vi "電池正負極設定.vi"() -> (3 "File Path":path=path "D:/battery/positive.txt")   [LabVIEW 2015]
uses:
  <vilib>/Utility/miscctls.llb/LVPointTypeDef.ctl
panel:
  in  "電池正負極陣列(輸入)":bool[](array[boolean])
  out "Enum":enum16{"一、讀取影像", "二、讀取設定檔", "三、寫入設定檔", "四、離開"}(ring)
  in  "離開":bool
  in  "寫入設定檔":bool
  in  "讀取設定檔":bool
  out "電池正負極陣列(輸出)":bool[](array[boolean])
  in  "電池正負極陣列叢集":T1
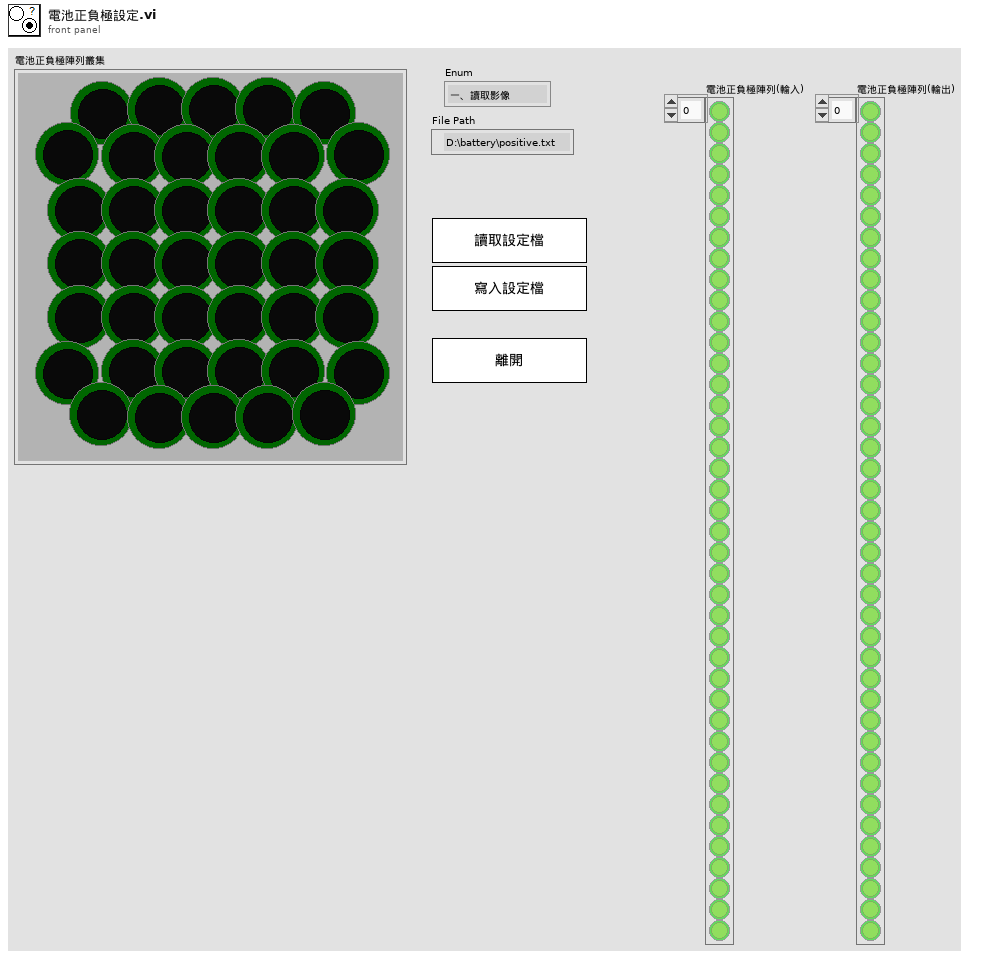
[diagram p1: front panel]
types:
  T1 = cluster{"Boolean":bool, "Boolean 2":bool, "Boolean 3":bool, "Boolean 4":bool, "Boolean 5":bool, "Boolean 6":bool, "Boolean 7":bool, "Boolean 8":bool, "Boolean 9":bool, "Boolean 10":bool, "Boolean 11":bool, "Boolean 12":bool, "Boolean 13":bool, "Boolean 14":bool, "Boolean 15":bool, "Boolean 16":bool, "Boolean 17":bool, "Boolean 18":bool, "Boolean 19":bool, "Boolean 20":bool, "Boolean 21":bool, "Boolean 22":bool, "Boolean 23":bool, "Boolean 24":bool, "Boolean 25":bool, "Boolean 26":bool, "Boolean 27":bool, "Boolean 28":bool, "Boolean 29":bool, "Boolean 30":bool, "Boolean 31":bool, "Boolean 32":bool, "Boolean 33":bool, "Boolean 34":bool, "Boolean 35":bool, "Boolean 36":bool, "Boolean 37":bool, "Boolean 38":bool, "Boolean 39":bool, "Boolean 40":bool}
  T2 = typedef "LVPointTypeDef.ctl" = cluster{"Horizontal":i16, "Vertical":i16}
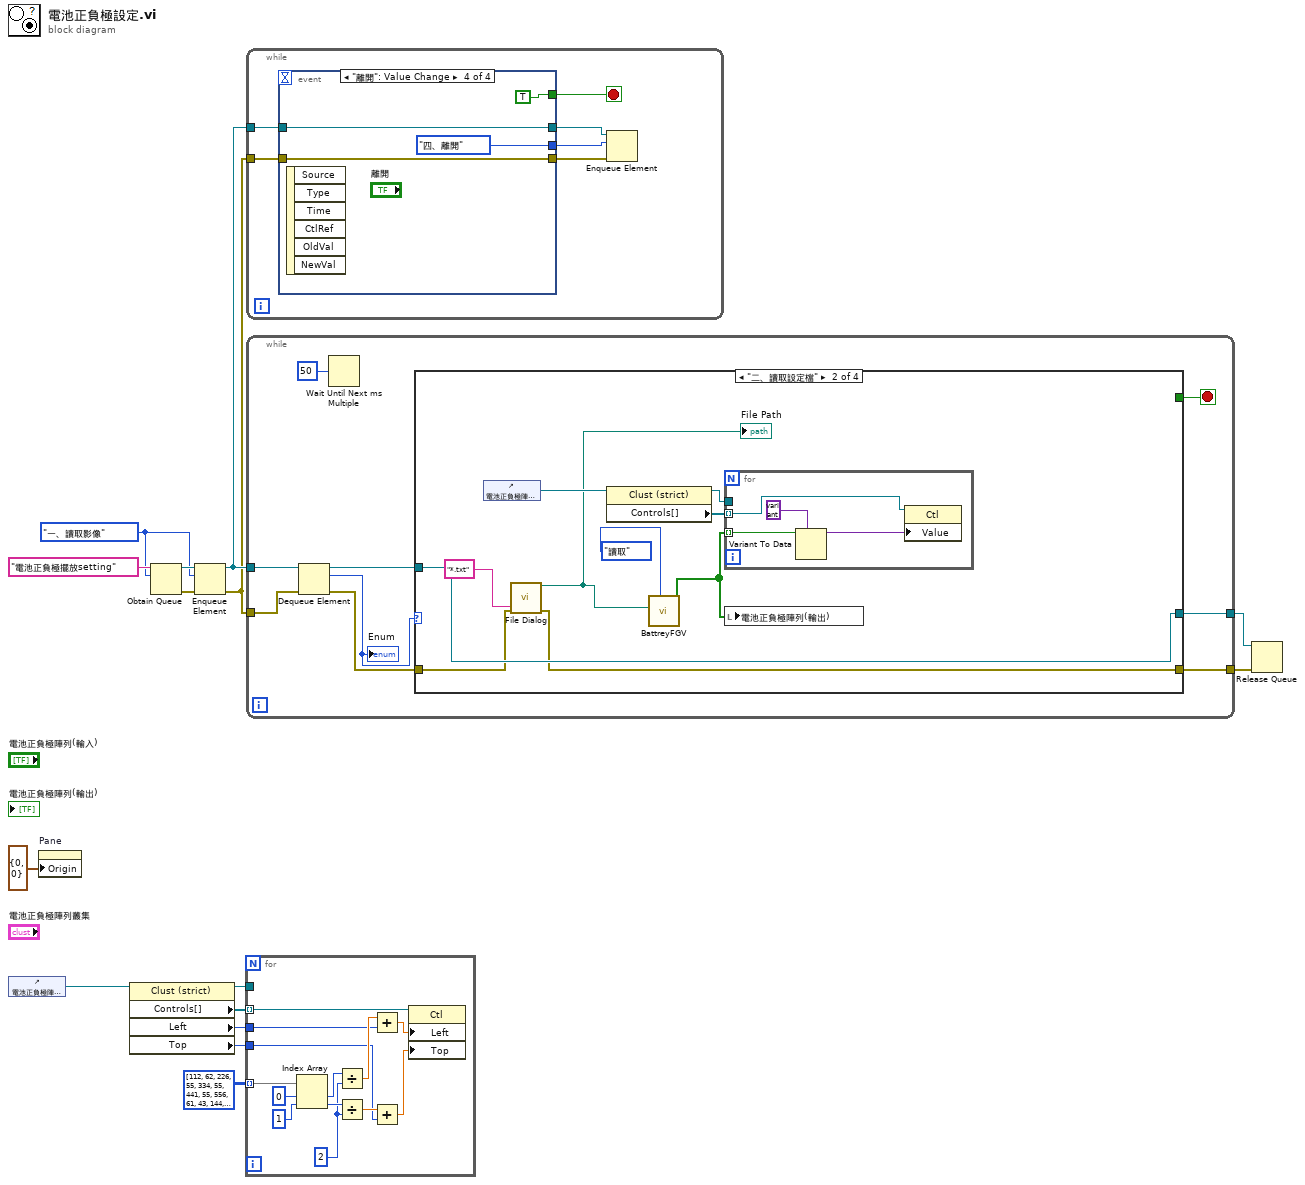
[diagram p0: block diagram]
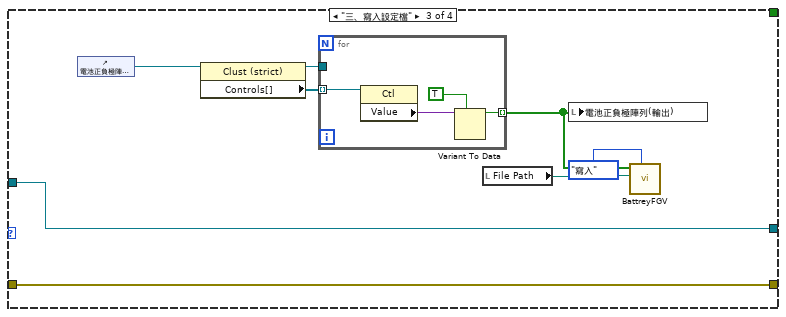
[diagram p3: hidden frame]
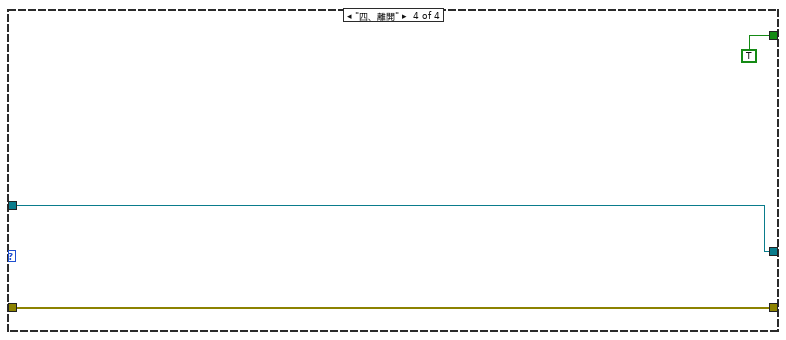
[diagram p4: hidden frame]
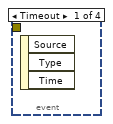
[diagram p5: hidden frame]
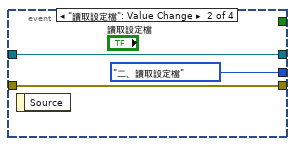
[diagram p6: hidden frame]
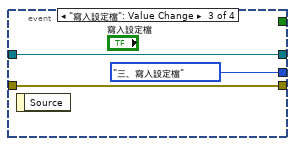
[diagram p7: hidden frame]
diagram:
  w6 = enum16{"一、讀取影像", "二、讀取設定檔", "三、寫入設定檔", "四、離開"}."一、讀取影像"
  n1 = control-ref of="電池正負極陣列叢集"() -> (w13:refnum<vi>)
  n2 = property on="Pane" class="Pane"("Origin"=T2 {"Horizontal"=0, "Vertical"=0}) -> ()  [unwired: 2 in, 2 out]
  n3 = property class="Clust (strict)"(reference=w13) -> (reference out=w15:refnum<vi>, "Controls[]"=w14:refnum<vi>[], "Left"=w11:i32, "Top"=w10:i32)  [unwired: 1 in, 1 out]
  n4 = Obtain Queue(name (unnamed)="電池正負極擺放setting", element data type=w6) -> (queue out=w8:refnum<queue>, error out=w7:errorcluster)  [unwired: 3 in, 1 out]
  n5 = Enqueue Element(queue=w8, element=w6, error in (no error)=w7) -> (queue out=w5:refnum<queue>, error out=w4:errorcluster)  [unwired: 1 in, 1 out]
  n6 = for {
    tunnel: w14 -> [w25] mode=indexing
    tunnel: w15 -> [_]
    tunnel: i32[][] [[112, 62], [226, 55], [334, 55], [441, 55], [556, 61], [43, 144], [173, 148], [280, 148], [387, 148], [494, 148], [624, 144], [66, 256], [173, 256], [280, 256], [387, 256], [494, 256], [602, 256], [66, 363], [173, 363], [280, 363], [387, 363], [494, 363], [602, 363], [66, 470], [173, 470], [280, 470], [387, 470], [494, 470], [602, 470], [43, 582], [173, 577], [280, 577], [387, 577], [494, 577], [624, 582], [111, 664], [226, 671], [334, 671], [441, 671], [556, 664]] ("array") -> [w28] mode=indexing
    tunnel: w11 -> [w17]
    tunnel: w10 -> [w16]
    w22 = 2 ("index")
    n7 = Index Array(array=w28, index #1=0 ("index"), index #2=1 ("index")) -> (element #1=w24:i32, element #2=w23:i32)
    n8 = Divide(x=w24, y=w22) -> (x/y=w20:dbl)
    n9 = Divide(x=w23, y=w22) -> (x/y=w21:dbl)
    n10 = Add(x=w20, y=w17) -> (x+y=w19:dbl)
    n11 = Add(x=w21, y=w16) -> (x+y=w18:dbl)
    n12 = property class="Ctl"(reference=w25, "Left"=w19, "Top"=w18) -> ()  [unwired: 1 in, 2 out]
  }
  n13 = while {
    tunnel: w5 -> [w33]
    tunnel: w4 -> [w32]
    stop <- w34 stop-if-true
    n14 = event shown="[3] \"離開\": Value Change" {
      selector: _ -> [_ _ _ _]
      dyn-events: _ -> [_ _ _ _]
      timeout: _ -> [_ _ _ _]
      tunnel: [_ _ _ TRUE] -> w34
      tunnel: w33 -> [_ w36 w39 w42]
      tunnel: w32 -> [_ w35 w38 w41]
      tunnel: [_ enum16{"一、讀取影像", "二、讀取設定檔", "三、寫入設定檔", "四、離開"}."二、讀取設定檔" enum16{"一、讀取影像", "二、讀取設定檔", "三、寫入設定檔", "四、離開"}."三、寫入設定檔" enum16{"一、讀取影像", "二、讀取設定檔", "三、寫入設定檔", "四、離開"}."四、離開"] -> w31
      tunnel: [_ w36 w39 w42] -> w30
      tunnel: [_ w35 w38 w41] -> w29
      event Timeout {
        n15 = event-data() -> ()  [unwired: 1 in, 3 out]
      }
      event "讀取設定檔": Value Change {
        n16 = event-data() -> ()  [unwired: 1 in, 1 out]
      }
      event "寫入設定檔": Value Change {
        n17 = event-data() -> ()  [unwired: 1 in, 1 out]
      }
      event "離開": Value Change {
        n18 = event-data() -> ()  [unwired: 1 in, 6 out]
      }
    }
    n19 = Enqueue Element(queue=w30, element=w31, error in (no error)=w29) -> ()  [unwired: 1 in, 3 out]
  }
  n20 = while {
    tunnel: w5 -> [w52]
    tunnel: w4 -> [w51]
    tunnel: [w47] -> w3
    tunnel: [w46] -> w2
    stop <- w45 stop-if-true
    n21 = Dequeue Element(queue=w52, error in (no error)=w51) -> (queue out=w49:refnum<queue>, element=w50:enum16{"一、讀取影像", "二、讀取設定檔", "三、寫入設定檔", "四、離開"}, error out=w48:errorcluster)  [unwired: 1 in, 1 out]
    "Enum" <- w50
    n22 = Wait Until Next ms Multiple(millisecond multiple=u32 50) -> ()  [unwired: 1 out]
    n23 = case shown="\"二、讀取設定檔\"" w50 {
      tunnel: [w55 w65 w77 w84] -> w47
      tunnel: w49 -> [w55 w65 w77 w84]
      tunnel: w48 -> [w54 w56 w76 w83]
      tunnel: [w54 w57 w76 w83] -> w46
      tunnel: [_ _ _ TRUE] -> w45
      frame "一、讀取影像", Default {
      }
      frame "二、讀取設定檔" {
        n24 = control-ref of="電池正負極陣列叢集"() -> (w62:refnum<vi>)
        n25 = call "File Dialog"("error in"=w56, "pattern (all files)"="*.txt") -> ("selected path"=w58:path, "error out"=w57:errorcluster)  [unwired: 10 in, 2 out]
        "File Path" <- w58
        n26 = property class="Clust (strict)"(reference=w62) -> (reference out=w64:refnum<vi>, "Controls[]"=w63:refnum<vi>[])  [unwired: 1 in, 1 out]
        n27 = call "BattreyFGV.vi"("Enum"=enum16{"初始化", "讀取", "寫入", "閒置"}."讀取", "File Path"=w58) -> ("電池正負極陣列(輸出)"=w61:bool[])  [unwired: 9 in]
        n28 = for {
          tunnel: w63 -> [w69] mode=indexing
          tunnel: w64 -> [_]
          tunnel: w61 -> [w67] mode=indexing
          n29 = Variant To Data(type=variant ("Value"), Variant=w67) -> (data=w66:variant)  [unwired: 1 in, 1 out]
          n30 = property class="Ctl"(reference=w69, "Value"=w66) -> ()  [unwired: 1 in, 2 out]
        }
        n31 = local write "電池正負極陣列(輸出)"(w61) -> ()
      }
      frame "三、寫入設定檔" {
        n32 = control-ref of="電池正負極陣列叢集"() -> (w73:refnum<vi>)
        n33 = property class="Clust (strict)"(reference=w73) -> (reference out=w74:refnum<vi>, "Controls[]"=w75:refnum<vi>[])  [unwired: 1 in, 1 out]
        n34 = for {
          tunnel: w75 -> [w81] mode=indexing
          tunnel: w74 -> [_]
          tunnel: [w80] -> w70 mode=indexing
          n35 = property class="Ctl"(reference=w81) -> ("Value"=w79:variant)  [unwired: 1 in, 2 out]
          n36 = Variant To Data(type=TRUE, Variant=w79) -> (data=w80:bool)  [unwired: 1 in, 1 out]
        }
        n37 = local read "File Path"() -> (w71:path)
        n38 = local write "電池正負極陣列(輸出)"(w70) -> ()
        n39 = call "BattreyFGV.vi"("Enum"=enum16{"初始化", "讀取", "寫入", "閒置"}."寫入", "File Path"=w71, "電池正負極陣列(輸入)"=w70) -> ()  [unwired: 8 in, 1 out]
      }
      frame "四、離開" {
      }
    }
  }
  n40 = Release Queue(queue=w3, error in (no error)=w2) -> ()  [unwired: 1 in, 3 out]
